vi "Teardown.vi"(8 "error in (no error)":errorcluster, 11 "Configuration File Interface Test In":refnum<class "Configuration File Base Interface Test.lvclass">) -> (0 "error out":errorcluster, 3 "Configuration File Interface Test Out":refnum<class "Configuration File Base Interface Test.lvclass">)   [LabVIEW 2020, in "Configuration File Base Interface Test.lvclass"]
uses:
  Configuration File Base Interface Test.lvclass
  Configuration File Base Interface Test.lvclass/Configuration File Base Interface Test.ctl
  Configuration Interface Test/Configuration Interface Test.lvclass
  Mock Configurable Base/Mock Configurable Base.lvclass
  Framework/Base/Base.lvclass
  C:/Git/triarc-framework/source/Framework Test/Configuration Interface Test/Configuration Interface Test.lvclass
  C:/Program Files (x86)/National Instruments/LabVIEW 2020/vi.lib/Astemes/LUnit/Test Case.lvclass
  C:/Git/triarc-framework/source/Framework Test/Configuration File Interface Test/Configuration File Base Interface Test.lvclass
  C:/Git/triarc-framework/source/Framework/Base/Base.lvclass
  C:/Git/triarc-framework/source/Framework/Configuration File/Configuration File.lvclass
  C:/Git/triarc-framework/source/Framework/Configuration/Configuration.lvclass
  C:/Git/triarc-framework/source/Framework Test/Mock Configurable Base/Mock Configurable Base.lvclass
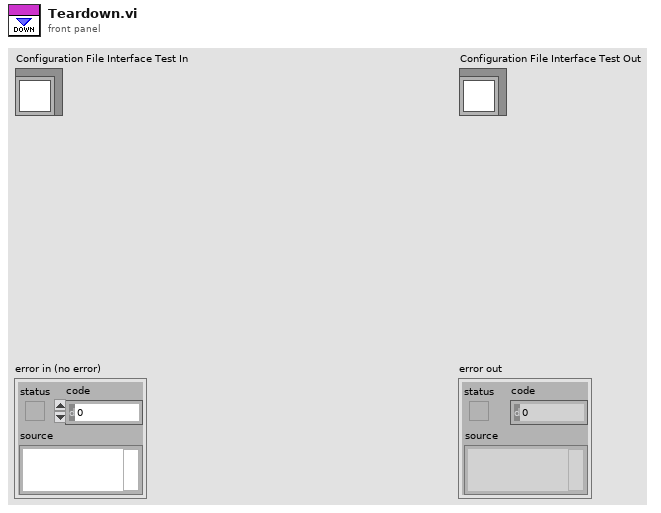
[diagram p1: front panel]
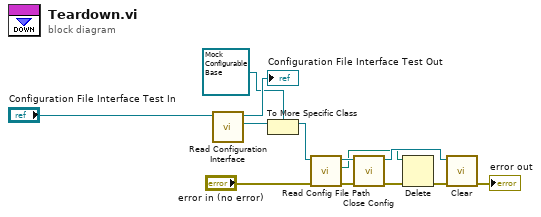
[diagram p0: block diagram]
diagram:
  n1 = call "Read Configuration Interface.vi"("Configuration Interface Test In"="Configuration File Interface Test In") -> ("Configuration"=w11:refnum<class "Configuration.lvclass">, "Configuration Interface Test Out"=→"Configuration File Interface Test Out":refnum<class "Configuration File Base Interface Test.lvclass">)  [unwired: 9 in]
  n2 = To More Specific Class(target class=refnum<class "Mock Configurable Base.lvclass"> refnum ("Mock Configurable.lvclass"), reference=w11) -> (specific class reference=w3:refnum<class "Mock Configurable Base.lvclass">)  [unwired: 1 in, 1 out]
  n3 = call "Read Config File Path.vi"("error in (no error)"="error in (no error)", "Base In"=w3) -> ("error out"=w4:errorcluster, "Config File Path"=w1:path, "Base Out"=w2:refnum<class "Mock Configurable Base.lvclass">)  [unwired: 7 in]
  n4 = call-dynamic "Close Config.vi"("error in (no error)"=w4, "Configuration File File In"=w2) -> ("error out"=w8:errorcluster, "Configuration File File Out"=w7:refnum<class "Mock Configurable Base.lvclass">)  [unwired: 8 in]
  n5 = Delete(path (use dialog)=w1, error in=w8) -> (error out=w9:errorcluster)  [unwired: 3 in, 2 out]
  n6 = call-dynamic "Clear.vi"("error in (no error)"=w9, "Base In"=w7) -> ("error out"=→"error out":errorcluster)  [unwired: 9 in]
